vi "加标回收启动 (子VI).vi"(11 "启动参数":T1(ring)=enum."CODCr") -> (0 "error out":T2={"status"=FALSE, "代码"=4, "source"=""} caption="错误输出" {"代码" items=["执行成功"=1, "执行失败，但不知道原因"=2, "命令请求条件错误"=3, "通讯超时"=4, "系统繁忙不能执行"=5, "系统故障"=6, "没有数据"=100]})   [LabVIEW 2016]
uses:
  PLC/PLC.lvlib
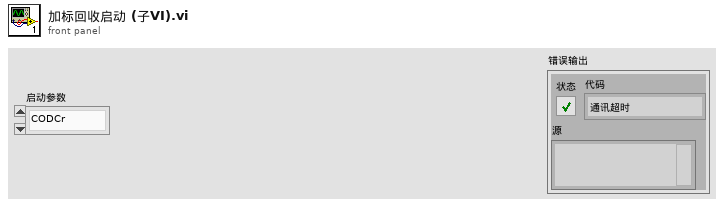
[diagram p1: front panel]
types:
  T1 = enum16{"未选择", "CODMn", "氨氮", "总磷", "总氮", "CODCr"}
  T2 = cluster{"status":bool, "代码":u16, "source":string}
  T3 = enum16{"空闲", "水样测试", "标样核查", "零点核查", "跨度核查", "空白测试", "平行样测试", "质控样", "空白校准", "标样校准", "加标回收"}
  T4 = enum16{"空闲", "水样测试", "标样核查", "零点核查", "跨度核查", "空白测试", "平行样测试", "加标回收", "空白校准", "标样校准", "初始化（清洗）"}
  T5 = cluster{"是否启用仪器":bool, "CODMn":cluster{"启动测量模式":cluster{"测量模式":enum16{"水样测量", "标样核查", "加标回收", "平行样", "校零", "校标"}}, "确定按钮":bool}, "启动模块":cluster{"氨氮":bool, "总磷":bool, "总氮":bool, "COD":bool}, "常规启动":bool, "直接启动":bool}
  T6 = cluster{"COD浓度（mg/L)":dbl, "水样启动时间":timestamp, "加标回收启动时间":timestamp, "CODMn工作状态":enum16{"空闲", "水样测试", "标样核查", "零点核查", "跨度核查", "空白测试", "平行样测试", "加标回收", "空白校准", "标样校准", "初始化（清洗）"}, "多列列表框":i32}
  T7 = cluster{"R0":i16, "R1":i16, "R2":i16, "R3":i16, "R4":i16, "R5":i16, "R6":i16, "R7":i16, "R8":i16, "R9":i16, "R10":i16, "R11":i16, "R12":i16, "R13":i16, "R14":i16, "R15":i16, "R16":i16, "R17":i16, "R18":i16, "R19":i16, "R20":i16, "R21":i16, "R22":i16, "R23":i16, "R24":i16, "R25":i16, "R26":i16, "R27":i16, "R28":i16, "R29":i16, "R30":i16, "R31":i16, "R32":i16, "R33":i16, "R34":i16}
  T8 = enum32{"Bad", "Idle", "Run top level", "Running"}
  T9 = cluster{"系统时间":timestamp, "工作状态":enum16{"空闲", "水样测试", "标样核查", "零点核查", "跨度核查", "空白测试", "平行样测试", "加标回收", "空白校准", "标样校准", "初始化（清洗）"}, "测量模式":enum16{"待机", "连续模式", "周期模式", "定点模式", "受控模式", "手动模式"}, "告警代码":u16, "故障代码":u16, "日志代码":u16, "软件版本":u16, "F0":sgl, "F1":sgl, "F2":sgl, "F3":sgl, "T":sgl, "H":sgl, "id":u16, "flowid":u16, "量程":u16, "总磷控温温度1":sgl, "营养盐控温温度2":sgl, "ADC":sgl}
  T10 = cluster{"系统时间":timestamp, "工作状态":u16, "测量模式":u16, "告警代码":u16, "故障代码":u16, "日志代码":u16, "软件版本":u16, "F0":sgl, "F1":sgl, "F2":sgl, "F3":sgl, "T":sgl, "H":sgl, "id":u16, "flowid":u16, "量程":u16}
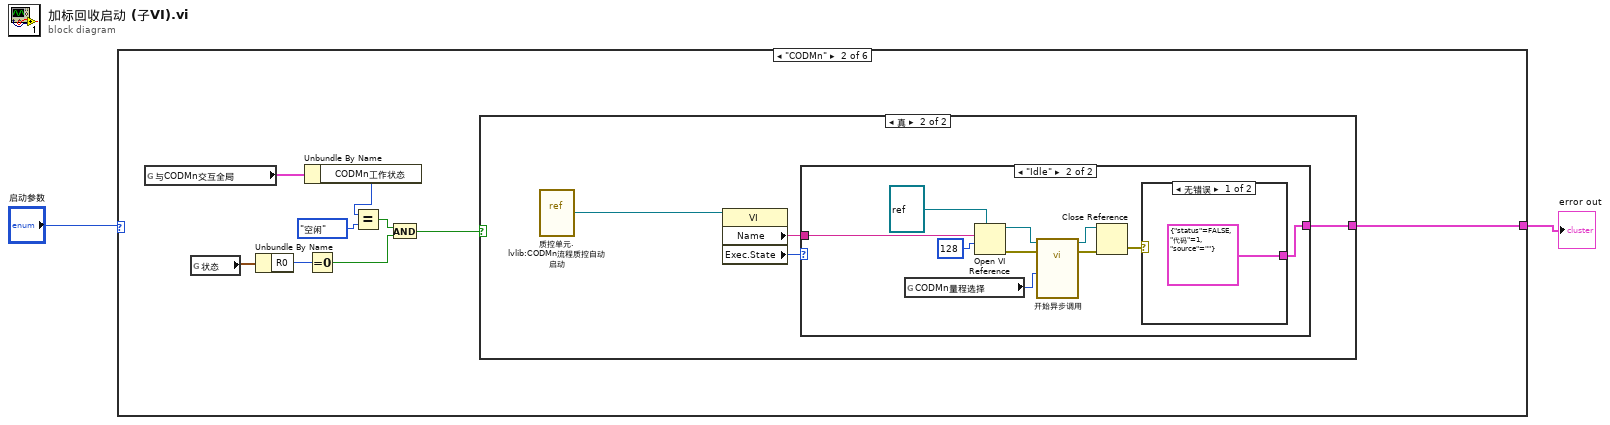
[diagram p0: block diagram]
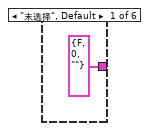
[diagram p2: hidden frame]
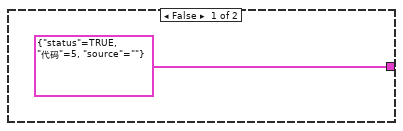
[diagram p3: hidden frame]
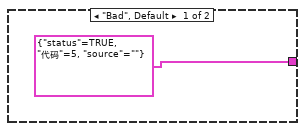
[diagram p4: hidden frame]
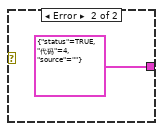
[diagram p5: hidden frame]
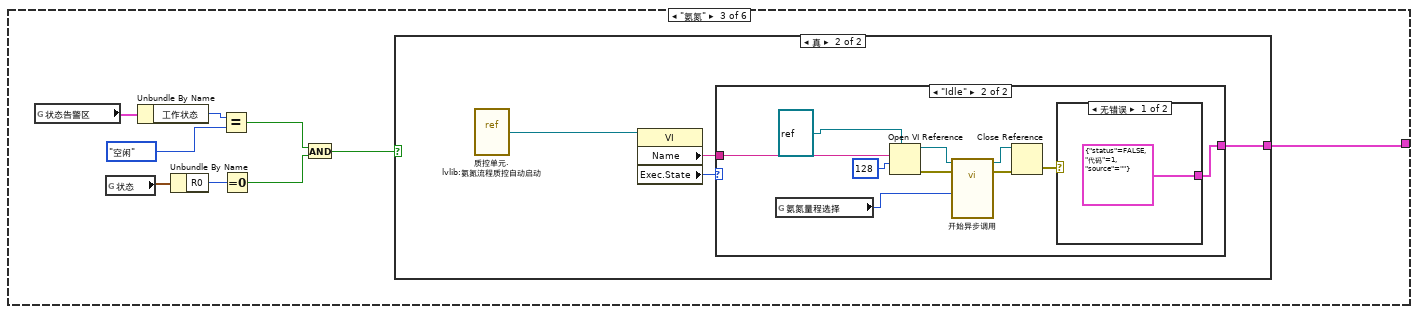
[diagram p6: hidden frame]
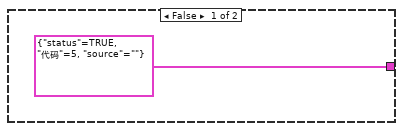
[diagram p7: hidden frame]
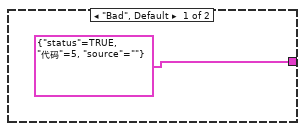
[diagram p8: hidden frame]
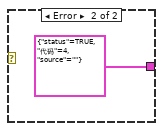
[diagram p9: hidden frame]
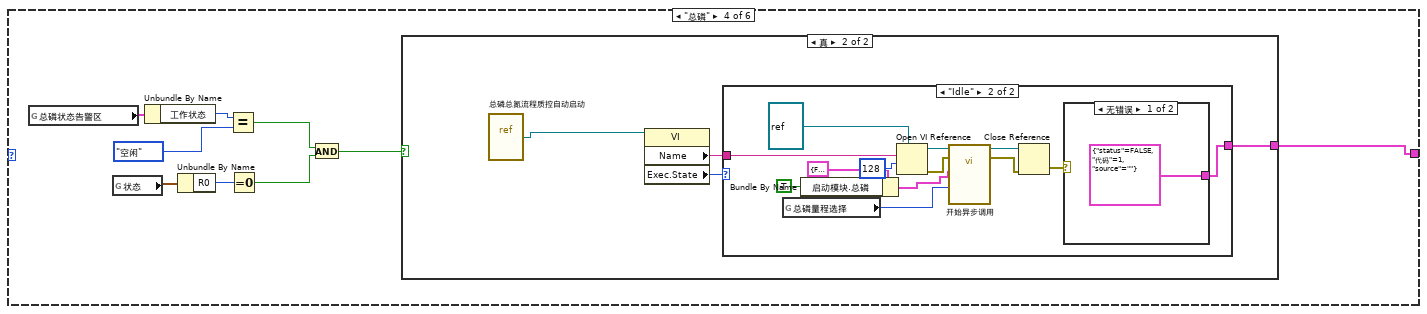
[diagram p10: hidden frame]
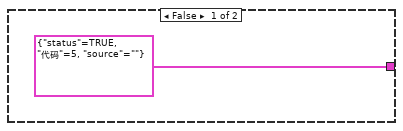
[diagram p11: hidden frame]
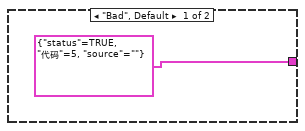
[diagram p12: hidden frame]
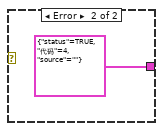
[diagram p13: hidden frame]
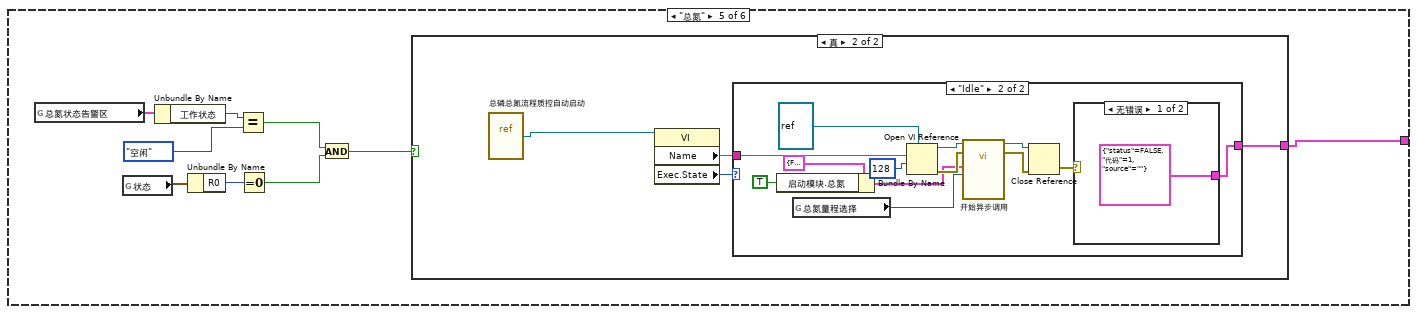
[diagram p14: hidden frame]
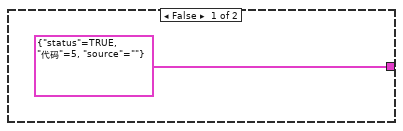
[diagram p15: hidden frame]
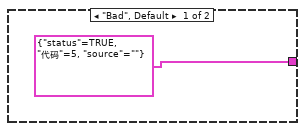
[diagram p16: hidden frame]
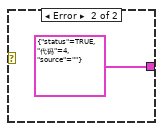
[diagram p17: hidden frame]
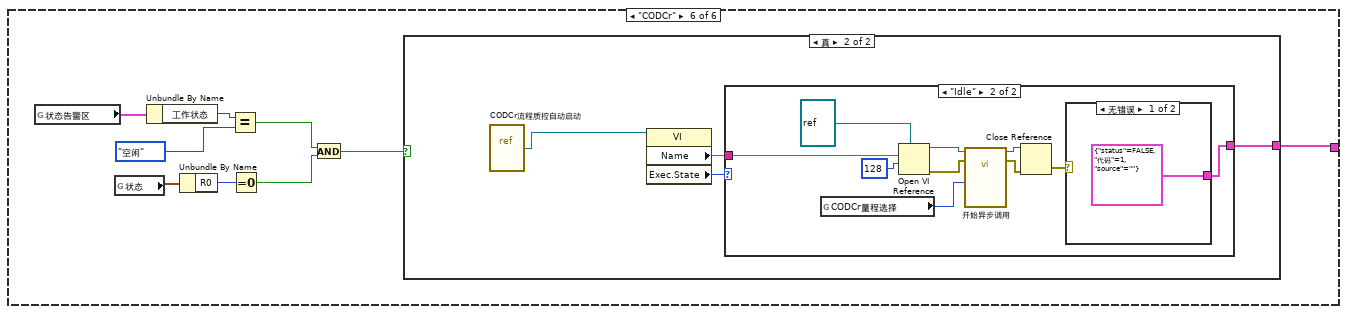
[diagram p18: hidden frame]
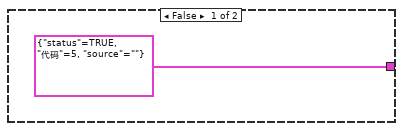
[diagram p19: hidden frame]
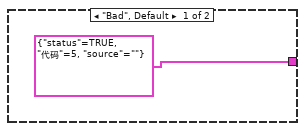
[diagram p20: hidden frame]
diagram:
  n1 = case shown="\"CODMn\"" "启动参数" {
    tunnel: [T2 {"status"=FALSE, "代码"=0, "source"=""} ("error out") w6 w35 w59 w88 w119] -> w1
    frame "未选择", Default {
    }
    frame "CODMn" {
      n2 = global read "modbus slave全局.vi" "与CODMn交互全局"() -> (w5:T6)
      n3 = global read "采配水全局变量.vi" "状态"() -> (w10:T7)
      n4 = Unbundle By Name(w10) -> ("R0"=w9:i16)
      n5 = Unbundle By Name(w5) -> ("CODMn工作状态"=w4:T4)
      n6 = Equal To 0?(x=w9) -> (x = 0?=w8:bool)
      n7 = Equal?(x=w4, y=T3."空闲") -> (x = y?=w11:bool)
      n8 = And(x=w11, y=w8) -> (x .and. y?=w7:bool)
      n9 = case shown="真" w7 {
        tunnel: [T2 {"status"=TRUE, "代码"=5, "source"=""} ("error out") w14] -> w6
        frame False {
        }
        frame True {
          n10 = vi-ref "质控单元.lvlib:CODMn流程质控自动启动.vi"() -> (w15:refnum<vi>)
          n11 = property class="VI"(reference=w15) -> ("Name"=w17:string, "Exec.State"=w16:T8)  [unwired: 1 in, 2 out]
          n12 = case shown="\"Idle\"" w16 {
            tunnel: w17 -> [_ w25]
            tunnel: [T2 {"status"=TRUE, "代码"=5, "source"=""} ("error out") w21] -> w14
            frame "Bad", Default {
            }
            frame "Idle" {
              n13 = global read "断电保存全局.vi" "CODMn量程选择"() -> (w19:enum32{"H", "L", "AUTO"})
              n14 = Open VI Reference(type specifier VI Refnum (for type only)=refnum<vi> refnum ("类型说明符VI引用句柄（仅用于类型）"), vi path=w25, options=128 ("选项")) -> (vi reference=w20:refnum<vi>, error out=w24:errorcluster)  [unwired: 3 in]
              n15 = call-by-ref "开始异步调用"(reference=w20, error in=w24, "CODMn量程切换"=w19) -> (reference out=w28:refnum<vi>, error out=w23:errorcluster)  [unwired: 10 in]
              n16 = Close Reference(reference=w28, error in (no error)=w23) -> (error out=w22:errorcluster)
              n17 = case shown="无错误" w22 {
                tunnel: [T2 {"status"=FALSE, "代码"=1, "source"=""} ("error out") T2 {"status"=TRUE, "代码"=4, "source"=""} ("error out")] -> w21
                frame No Error {
                }
                frame Error {
                }
              }
            }
          }
        }
      }
    }
    frame "氨氮" {
      n18 = global read "VAR氨氮全局变量.vi" "状态告警区"() -> (w34:T9)
      n19 = global read "采配水全局变量.vi" "状态"() -> (w39:T7)
      n20 = Unbundle By Name(w34) -> ("工作状态"=w33:T4)
      n21 = Unbundle By Name(w39) -> ("R0"=w38:i16)
      n22 = Equal?(x=w33, y=T4."空闲") -> (x = y?=w31:bool)
      n23 = Equal To 0?(x=w38) -> (x = 0?=w37:bool)
      n24 = And(x=w31, y=w37) -> (x .and. y?=w36:bool)
      n25 = case shown="真" w36 {
        tunnel: [T2 {"status"=TRUE, "代码"=5, "source"=""} ("error out") w42] -> w35
        frame False {
        }
        frame True {
          n26 = vi-ref "质控单元.lvlib:氨氮流程质控自动启动.vi"() -> (w41:refnum<vi>)
          n27 = property class="VI"(reference=w41) -> ("Name"=w44:string, "Exec.State"=w43:T8)  [unwired: 1 in, 2 out]
          n28 = case shown="\"Idle\"" w43 {
            tunnel: w44 -> [_ w52]
            tunnel: [T2 {"status"=TRUE, "代码"=5, "source"=""} ("error out") w48] -> w42
            frame "Bad", Default {
            }
            frame "Idle" {
              n29 = global read "断电保存全局.vi" "氨氮量程选择"() -> (w46:enum32{"H", "L", "AUTO"})
              n30 = Open VI Reference(type specifier VI Refnum (for type only)=refnum<vi> refnum ("类型说明符VI引用句柄（仅用于类型）"), vi path=w52, options=128 ("选项")) -> (vi reference=w55:refnum<vi>, error out=w51:errorcluster)  [unwired: 3 in]
              n31 = call-by-ref "开始异步调用"(reference=w55, error in=w51, "氨氮量程切换"=w46) -> (reference out=w54:refnum<vi>, error out=w50:errorcluster)  [unwired: 11 in]
              n32 = Close Reference(reference=w54, error in (no error)=w50) -> (error out=w49:errorcluster)
              n33 = case shown="无错误" w49 {
                tunnel: [T2 {"status"=FALSE, "代码"=1, "source"=""} ("error out") T2 {"status"=TRUE, "代码"=4, "source"=""} ("error out")] -> w48
                frame No Error {
                }
                frame Error {
                }
              }
            }
          }
        }
      }
    }
    frame "总磷" {
      n34 = global read "VAR总磷总氮全局变量.vi" "总磷状态告警区"() -> (w58:T9)
      n35 = global read "采配水全局变量.vi" "状态"() -> (w66:T7)
      n36 = Unbundle By Name(w58) -> ("工作状态"=w62:T4)
      n37 = Unbundle By Name(w66) -> ("R0"=w65:i16)
      n38 = Equal?(x=w62, y=T4."空闲") -> (x = y?=w60:bool)
      n39 = Equal To 0?(x=w65) -> (x = 0?=w64:bool)
      n40 = And(x=w60, y=w64) -> (x .and. y?=w63:bool)
      n41 = case shown="真" w63 {
        tunnel: [T2 {"status"=TRUE, "代码"=5, "source"=""} ("error out") w69] -> w59
        frame False {
        }
        frame True {
          n42 = vi-ref "总磷总氮流程质控自动启动.vi"() -> (w68:refnum<vi>)
          n43 = property class="VI"(reference=w68) -> ("Name"=w71:string, "Exec.State"=w70:T8)  [unwired: 1 in, 2 out]
          n44 = case shown="\"Idle\"" w70 {
            tunnel: w71 -> [_ w84]
            tunnel: [T2 {"status"=TRUE, "代码"=5, "source"=""} ("error out") w81] -> w69
            frame "Bad", Default {
            }
            frame "Idle" {
              n45 = global read "断电保存全局.vi" "总磷量程选择"() -> (w76:enum32{"H", "L", "AUTO"})
              n46 = Bundle By Name(cluster=T5 {"是否启用仪器"=FALSE, "CODMn"={"启动测量模式"={"测量模式"=enum."水样测量"}, "确定按钮"=FALSE}, "启动模块"={"氨氮"=FALSE, "总磷"=FALSE, "总氮"=FALSE, "COD"=FALSE}, "常规启动"=FALSE, "直接启动"=FALSE} ("参数"), "启动模块.总磷"=TRUE) -> (w73:T5)
              n47 = Open VI Reference(type specifier VI Refnum (for type only)=refnum<vi> refnum ("类型说明符VI引用句柄（仅用于类型）"), vi path=w84, options=128 ("选项")) -> (vi reference=w79:refnum<vi>, error out=w78:errorcluster)  [unwired: 3 in]
              n48 = call-by-ref "开始异步调用"(reference=w79, error in=w78, "总磷量程切换"=w76, "参数"=w73) -> (reference out=w77:refnum<vi>, error out=w83:errorcluster)  [unwired: 10 in]
              n49 = Close Reference(reference=w77, error in (no error)=w83) -> (error out=w82:errorcluster)
              n50 = case shown="无错误" w82 {
                tunnel: [T2 {"status"=FALSE, "代码"=1, "source"=""} ("error out") T2 {"status"=TRUE, "代码"=4, "source"=""} ("error out")] -> w81
                frame No Error {
                }
                frame Error {
                }
              }
            }
          }
        }
      }
    }
    frame "总氮" {
      n51 = global read "VAR总磷总氮全局变量.vi" "总氮状态告警区"() -> (w89:T9)
      n52 = global read "采配水全局变量.vi" "状态"() -> (w96:T7)
      n53 = Unbundle By Name(w89) -> ("工作状态"=w92:T4)
      n54 = Unbundle By Name(w96) -> ("R0"=w95:i16)
      n55 = Equal?(x=w92, y=T4."空闲") -> (x = y?=w90:bool)
      n56 = Equal To 0?(x=w95) -> (x = 0?=w94:bool)
      n57 = And(x=w90, y=w94) -> (x .and. y?=w93:bool)
      n58 = case shown="真" w93 {
        tunnel: [T2 {"status"=TRUE, "代码"=5, "source"=""} ("error out") w99] -> w88
        frame False {
        }
        frame True {
          n59 = vi-ref "总磷总氮流程质控自动启动.vi"() -> (w98:refnum<vi>)
          n60 = property class="VI"(reference=w98) -> ("Name"=w101:string, "Exec.State"=w100:T8)  [unwired: 1 in, 2 out]
          n61 = case shown="\"Idle\"" w100 {
            tunnel: w101 -> [_ w114]
            tunnel: [T2 {"status"=TRUE, "代码"=5, "source"=""} ("error out") w112] -> w99
            frame "Bad", Default {
            }
            frame "Idle" {
              n62 = Bundle By Name(cluster=T5 {"是否启用仪器"=FALSE, "CODMn"={"启动测量模式"={"测量模式"=enum."水样测量"}, "确定按钮"=FALSE}, "启动模块"={"氨氮"=FALSE, "总磷"=FALSE, "总氮"=FALSE, "COD"=FALSE}, "常规启动"=FALSE, "直接启动"=FALSE} ("参数"), "启动模块.总氮"=TRUE) -> (w103:T5)
              n63 = global read "断电保存全局.vi" "总氮量程选择"() -> (w108:enum32{"H", "L", "AUTO"})
              n64 = Open VI Reference(type specifier VI Refnum (for type only)=refnum<vi> refnum ("类型说明符VI引用句柄（仅用于类型）"), vi path=w114, options=128 ("选项")) -> (vi reference=w110:refnum<vi>, error out=w109:errorcluster)  [unwired: 3 in]
              n65 = call-by-ref "开始异步调用"(reference=w110, error in=w109, "总氮量程切换"=w108, "参数"=w103) -> (reference out=w107:refnum<vi>, error out=w106:errorcluster)  [unwired: 10 in]
              n66 = Close Reference(reference=w107, error in (no error)=w106) -> (error out=w113:errorcluster)
              n67 = case shown="无错误" w113 {
                tunnel: [T2 {"status"=FALSE, "代码"=1, "source"=""} ("error out") T2 {"status"=TRUE, "代码"=4, "source"=""} ("error out")] -> w112
                frame No Error {
                }
                frame Error {
                }
              }
            }
          }
        }
      }
    }
    frame "CODCr" {
      n68 = global read "CODcr全局变量.vi" "状态告警区"() -> (w118:T10)
      n69 = global read "采配水全局变量.vi" "状态"() -> (w126:T7)
      n70 = Unbundle By Name(w118) -> ("工作状态"=w122:u16)
      n71 = Unbundle By Name(w126) -> ("R0"=w125:i16)
      n72 = Equal?(x=w122, y=T4."空闲") -> (x = y?=w120:bool)
      n73 = Equal To 0?(x=w125) -> (x = 0?=w124:bool)
      n74 = And(x=w120, y=w124) -> (x .and. y?=w123:bool)
      n75 = case shown="真" w123 {
        tunnel: [T2 {"status"=TRUE, "代码"=5, "source"=""} ("error out") w129] -> w119
        frame False {
        }
        frame True {
          n76 = vi-ref "CODCr流程质控自动启动.vi"() -> (w128:refnum<vi>)
          n77 = property class="VI"(reference=w128) -> ("Name"=w131:string, "Exec.State"=w130:T8)  [unwired: 1 in, 2 out]
          n78 = case shown="\"Idle\"" w130 {
            tunnel: w131 -> [_ w141]
            tunnel: [T2 {"status"=TRUE, "代码"=5, "source"=""} ("error out") w139] -> w129
            frame "Bad", Default {
            }
            frame "Idle" {
              n79 = global read "断电保存全局.vi" "CODCr量程选择"() -> (w136:enum32{"H", "L", "AUTO"})
              n80 = Open VI Reference(type specifier VI Refnum (for type only)=refnum<vi> refnum ("类型说明符VI引用句柄（仅用于类型）"), vi path=w141, options=128 ("选项")) -> (vi reference=w137:refnum<vi>, error out=w135:errorcluster)  [unwired: 3 in]
              n81 = call-by-ref "开始异步调用"(reference=w137, error in=w135, "CODCr量程切换"=w136) -> (reference out=w134:refnum<vi>, error out=w133:errorcluster)  [unwired: 10 in]
              n82 = Close Reference(reference=w134, error in (no error)=w133) -> (error out=w140:errorcluster)
              n83 = case shown="无错误" w140 {
                tunnel: [T2 {"status"=FALSE, "代码"=1, "source"=""} ("error out") T2 {"status"=TRUE, "代码"=4, "source"=""} ("error out")] -> w139
                frame No Error {
                }
                frame Error {
                }
              }
            }
          }
        }
      }
    }
  }
  "error out" <- w1
